vi "Subscribe JSON.vi"(7 "Options":string, 8 "error in (no error)":errorcluster, 9 "Time out ms (1000)":i32=1000, 10 "Topic":string, 11 "WAMP Client in":refnum<class "WAMP Client.lvclass">) -> (0 "error out":errorcluster, 1 "Publication Received Notifier":refnum<notifier>, 2 "Publication Received Event":refnum<user-event>, 3 "WAMP Client out":refnum<class "WAMP Client.lvclass">, 5 "WAMP Error":T1={"URI"="", "Arguments Payload"="", "ArgumentKw Payload"="{}", "Details"="{}", "Associated LabVIEW Error"={"status"=FALSE, "code"=0, "source"=""}})   [LabVIEW 2020, in "wamplv.lvlib" / "WAMP Client.lvclass"]
uses:
  WAMP Client.lvclass
  WAMP Client.lvclass/WAMP Client.ctl
  5ceb9273-3c02-4cd5-9f1b-4889f58c0d6e.vi
  Private/Message loop classes/Subscription details/SubscriptionDetailsParent/SubscriptionDetailsParent.lvclass
  C:/local/wamplv/Private/Message loop classes/Subscription details/SubscriptionDetailsParent/SubscriptionDetailsParent.lvclass
  C:/local/wamplv/Private/Requests/IContainersNotiferOrEvents/IContainersNotiferOrEvents.lvclass
  Private/TypeDef/EVENT payload (JSON).ctl
  wamplv.lvlib
  TypeDefs/Error or abort detail (JSON).ctl
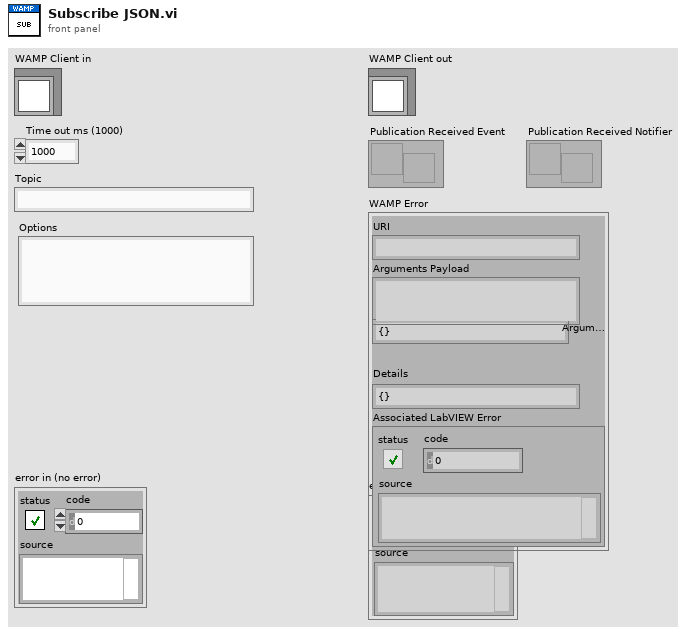
[diagram p1: front panel]
types:
  T1 = typedef "wamplv.lvlib/Error or abort detail (JSON).ctl" = cluster{"URI":string, "Arguments Payload":string, "ArgumentKw Payload":string, "Details":string, "Associated LabVIEW Error":errorcluster}
  T2 = typedef "wamplv.lvlib/Subscribe result (JSON).ctl" = cluster{"Publication Received Event":refnum<user-event>, "Publication Received Notifier":refnum<notifier>, "Sucess or error (JSON)":T3}
  T3 = typedef "wamplv.lvlib/Success or error (JSON).ctl" = cluster{"Success?":bool, "URI":string, "Error/Abort details (JSON)":T1}
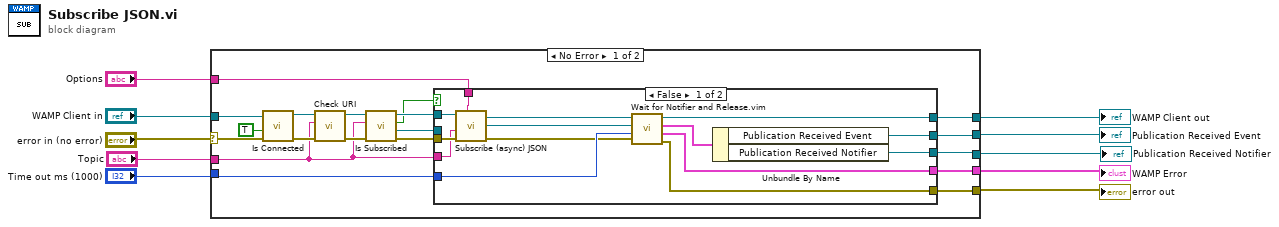
[diagram p0: block diagram]
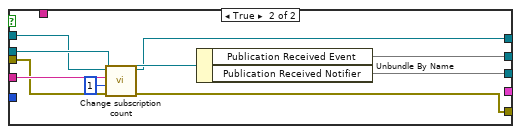
[diagram p2: hidden frame]
diagram:
  n1 = case shown="No Error" "error in (no error)" {
    selector: "error in (no error)" -> [w23 w53]
    tunnel: [w29 w53] -> w10
    tunnel: [w28 w54] -> w9
    tunnel: "Time out ms (1000)" -> [w27 _]
    tunnel: [w26 _] -> w7
    tunnel: [w25 _] -> w6
    tunnel: "WAMP Client in" -> [w24 w54]
    tunnel: "Topic" -> [w12 _]
    tunnel: "Options" -> [w19 _]
    tunnel: [w18 _] -> w1
    frame No Error {
      n2 = call "Is Connected.vi"("error in"=w23, "Raise error if not connected"=TRUE, "WAMP Client in"=w24) -> ("error out"=w21:errorcluster, "WAMP Client out"=w20:refnum<class "WAMP Client.lvclass">)  [unwired: 6 in, 1 out]
      n3 = call "Check URI.vi"("error in (no error)"=w21, "URI"=w12, "WAMP Client in"=w20) -> ("error out"=w15:errorcluster, "WAMP Client out"=w16:refnum<class "WAMP Client.lvclass">)  [unwired: 5 in, 2 out]
      n4 = call-dynamic "Is Subscribed.vi"("error in (no error)"=w15, "Topic"=w12, "WAMP Client in"=w16) -> ("error out"=w13:errorcluster, "SubscriptionDetailsParent out"=w11:refnum<class "SubscriptionDetailsParent.lvclass">, "Found?"=w14:bool, "WAMP Client out"=w17:refnum<class "WAMP Client.lvclass">)  [unwired: 5 in]
      n5 = case shown="False" w14 {
        tunnel: [w43 w46] -> w29
        tunnel: [w42 w44] -> w28
        tunnel: w27 -> [w41 _]
        tunnel: [w40 _] -> w26
        tunnel: [w39 w51] -> w25
        tunnel: w19 -> [w38 _]
        tunnel: [w33 w50] -> w18
        tunnel: w17 -> [w32 w49]
        tunnel: w13 -> [w31 w47]
        tunnel: w12 -> [w30 w48]
        tunnel: w11 -> [_ w52]
        frame False {
          n6 = call-dynamic "Subscribe (async) JSON.vi"("Options"=w38, "error in (no error)"=w31, "Topic"=w30, "WAMP Client in"=w32) -> ("error out"=w37:errorcluster, "notifier out"=w36:refnum<notifier>, "WAMP Client out"=w35:refnum<class "WAMP Client.lvclass">)  [unwired: 5 in]
          n7 = call "Wait for Notifier and Release.vim"("error in (no error)"=w37, "timeout in ms (0)"=w41, "Notifier in"=w36, "WAMP Client in"=w35) -> ("error out"=w43:errorcluster, "WAMP Error"=w40:T1, "Data"=w34:T2, "WAMP Client out"=w42:refnum<class "WAMP Client.lvclass">)  [unwired: 4 in]
          n8 = Unbundle By Name(w34) -> ("Publication Received Event"=w39:refnum<user-event>, "Publication Received Notifier"=w33:refnum<notifier>)
        }
        frame True {
          n9 = call-dynamic "Change subscription count.vi"("error in (no error)"=w47, "Count change"=i64 1, "Topic"=w48, "WAMP Client in"=w49) -> ("error out"=w46:errorcluster, "WAMP Client out"=w44:refnum<class "WAMP Client.lvclass">)  [unwired: 6 in]
          n10 = Unbundle By Name(w52) -> ("Publication Received Event"=w51, "Publication Received Notifier"=w50)
        }
      }
    }
    frame Error {
    }
  }
  "error out" <- w10
  "WAMP Client out" <- w9
  "Publication Received Event" <- w6
  "WAMP Error" <- w7
  "Publication Received Notifier" <- w1
